vi "test_MSS simulated scope.vi"(8 "Error In":errorcluster) -> (0 "Error Out":errorcluster)   [LabVIEW 2023]
uses:
  Measure and Stimulus Subsystems/Measure and Stimulus Subsystems.lvclass
panel:
  out "Powersensor Chart":waveform(dbl)(graph)
  in  "Stop":bool
  out "Photosensor Chart":waveform(dbl)(graph)
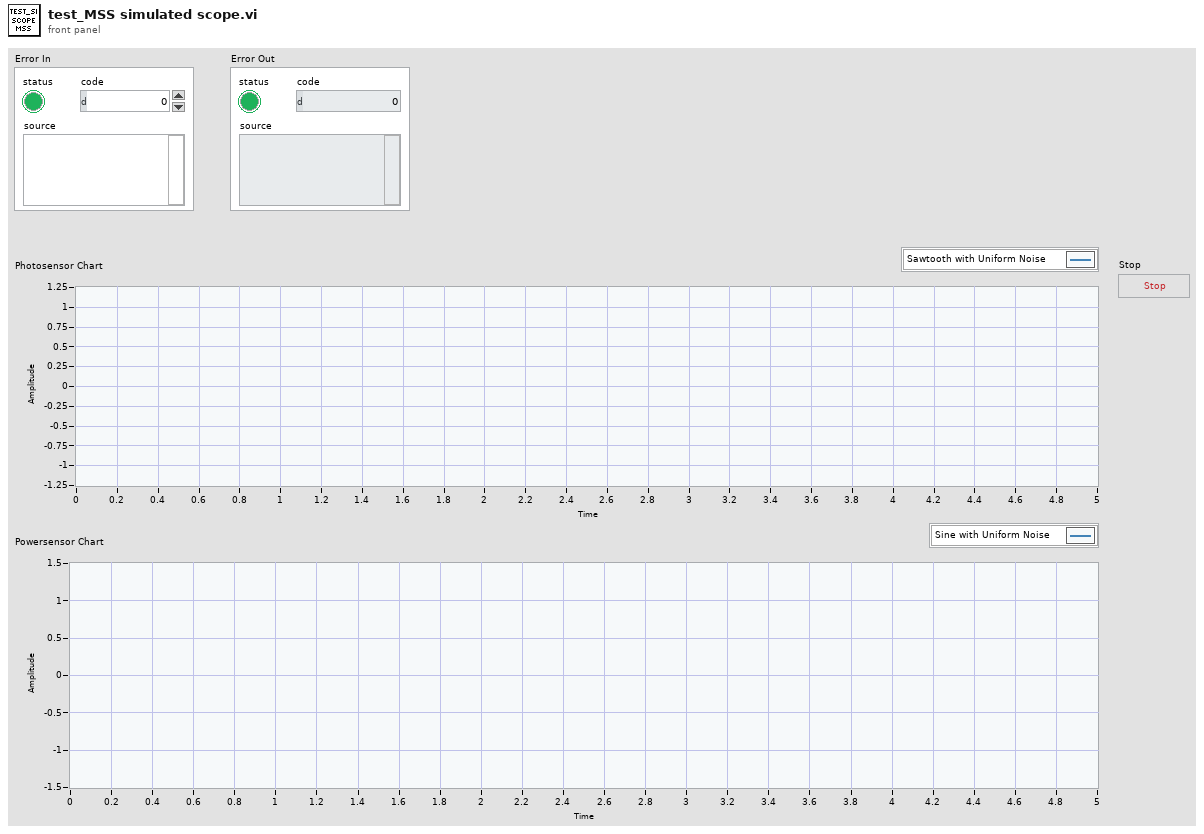
[diagram p1: front panel]
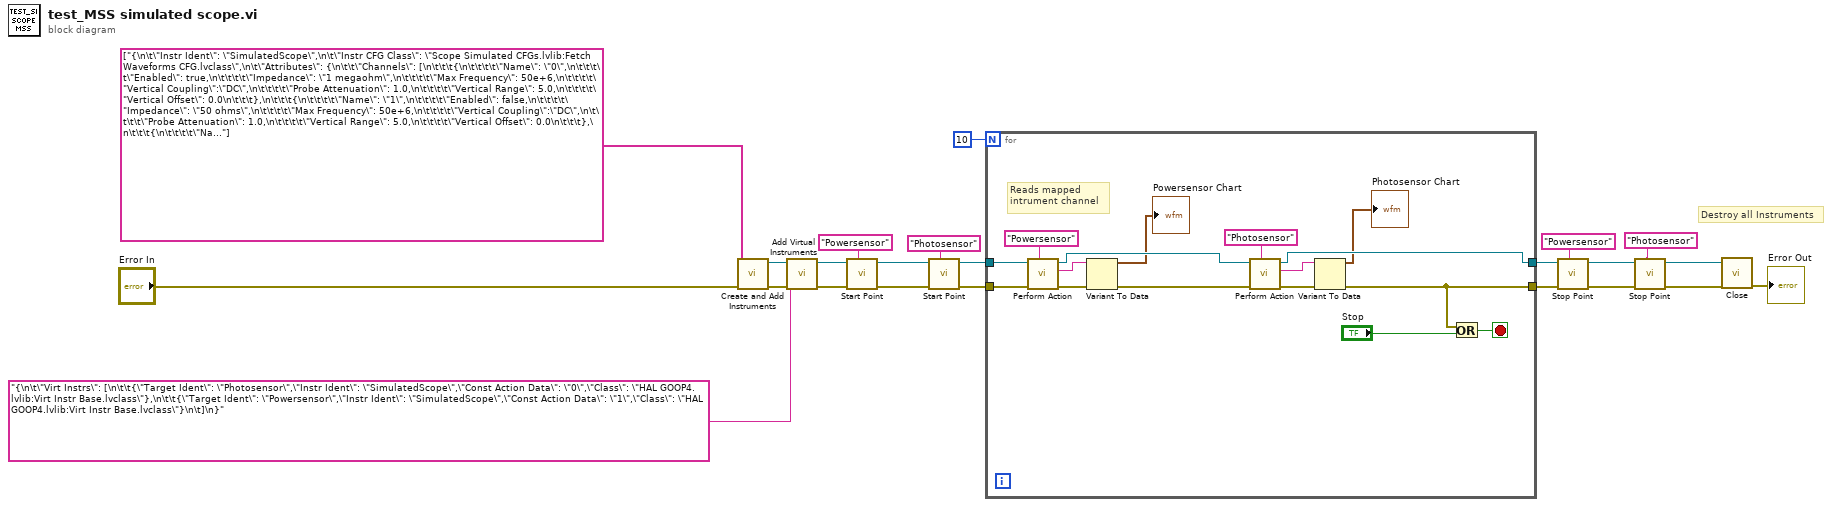
[diagram p0: block diagram]
diagram:
  # "Destroy all Instruments"
  n1 = call "Create and Add Instruments.vi"("Error In"="Error In", "Physical Intr CFGs"=string[] ["{\n\t\"Instr Ident\": \"SimulatedScope\",\n\t\"Instr CFG Class\": \"Scope Simulated CFGs.lvlib:Fetch Waveforms CFG.lvclass\",\n\t\"Attributes\": {\n\t\t\"Channels\": [\n\t\t\t{\n\t\t\t\t\"Name\": \"0\",\n\t\t\t\t\"Enabled\": true,\n\t\t\t\t\"Impedance\": \"1 megaohm\",\n\t\t\t\t\"Max Frequency\": 50e+6,\n\t\t\t\t\"Vertical Coupling\":\"DC\",\n\t\t\t\t\"Probe Attenuation\": 1.0,\n\t\t\t\t\"Vertical Range\": 5.0,\n\t\t\t\t\"Vertical Offset\": 0.0\n\t\t\t},\n\t\t\t{\n\t\t\t\t\"Name\": \"1\",\n\t\t\t\t\"Enabled\": false,\n\t\t\t\t\"Impedance\": \"50 ohms\",\n\t\t\t\t\"Max Frequency\": 50e+6,\n\t\t\t\t\"Vertical Coupling\":\"DC\",\n\t\t\t\t\"Probe Attenuation\": 1.0,\n\t\t\t\t\"Vertical Range\": 5.0,\n\t\t\t\t\"Vertical Offset\": 0.0\n\t\t\t},\n\t\t\t{\n\t\t\t\t\"Name\": \"2\",\n\t\t\t\t\"Enabled\": false,\n\t\t\t\t\"Impedance\": \"50 ohms\",\n\t\t\t\t\"Max Frequency\": 50e+6,\n\t\t\t\t\"Vertical Coupling\":\"DC\",\n\t\t\t\t\"Probe Attenuation\": 1.0,\n\t\t\t\t\"Vertical Range\": 5.0,\n\t\t\t\t\"Vertical Offset\": 0.0\n\t\t\t},\n\t\t\t{\n\t\t\t\t\"Name\": \"3\",\n\t\t\t\t\"Enabled\": true,\n\t\t\t\t\"Impedance\": \"50 ohms\",\n\t\t\t\t\"Max Frequency\": 50e+6,\n\t\t\t\t\"Vertical Coupling\":\"DC\",\n\t\t\t\t\"Probe Attenuation\": 1.0,\n\t\t\t\t\"Vertical Range\": 1.4,\n\t\t\t\t\"Vertical Offset\": 0.0\n\t\t\t},\n\t\t\t{\n\t\t\t\t\"Name\": \"4\",\n\t\t\t\t\"Enabled\": false,\n\t\t\t\t\"Impedance\": \"50 ohms\",\n\t\t\t\t\"Max Frequency\": 50e+6,\n\t\t\t\t\"Vertical Coupling\":\"DC\",\n\t\t\t\t\"Probe Attenuation\": 1.0,\n\t\t\t\t\"Vertical Range\": 5.0,\n\t\t\t\t\"Vertical Offset\": 0.0\n\t\t\t},\n\t\t\t{\n\t\t\t\t\"Name\": \"5\",\n\t\t\t\t\"Enabled\": false,\n\t\t\t\t\"Impedance\": \"50 ohms\",\n\t\t\t\t\"Max Frequency\": 50e+6,\n\t\t\t\t\"Vertical Coupling\":\"DC\",\n\t\t\t\t\"Probe Attenuation\": 1.0,\n\t\t\t\t\"Vertical Range\": 5.0,\n\t\t\t\t\"Vertical Offset\": 0.0\n\t\t\t},\n\t\t\t{\n\t\t\t\t\"Name\": \"6\",\n\t\t\t\t\"Enabled\": false,\n\t\t\t\t\"Impedance\": \"50 ohms\",\n\t\t\t\t\"Max Frequency\": 50e+6,\n\t\t\t\t\"Vertical Coupling\":\"DC\",\n\t\t\t\t\"Probe Attenuation\": 1.0,\n\t\t\t\t\"Vertical Range\": 5.0,\n\t\t\t\t\"Vertical Offset\": 0.0\n\t\t\t},\n\t\t\t{\n\t\t\t\t\"Name\": \"7\",\n\t\t\t\t\"Enabled\": false,\n\t\t\t\t\"Impedance\": \"50 ohms\",\n\t\t\t\t\"Max Frequency\": 50e+6,\n\t\t\t\t\"Vertical Coupling\":\"DC\",\n\t\t\t\t\"Probe Attenuation\": 1.0,\n\t\t\t\t\"Vertical Range\": 5.0,\n\t\t\t\t\"Vertical Offset\": 0.0\n\t\t\t}\n\t\t],\n\t\t\"Horizontal\": {\n\t\t\t\"Enforce Realtime\": true,\n\t\t\t\"Number of Records\": 1,\n\t\t\t\"Min Sample Rate\": 1e+5,\n\t\t\t\"Reference Position\":50, //percent\n\t\t\t\"Min Record Length\":1e+3\n\t\t},\n\t\t\"Acquire\": {\n\t\t\t\"Type\": \"Normal\",\n\t\t\t\"NumSamples\": 1e+3,\n\t\t\t\"Fetch Relative To\": \"Read Pointer\"\n\t\t},\n\t\t\"Export Signal\": {\n\t\t\t\"Signal Identifier\": \"None\",\n\t\t\t\"Signal\": \"None\",\n\t\t\t\"Output Terminal\": \"None\"\n\t\t},\n\t\t\"Trigger\": {\n\t\t\t\"Type\": \"Immediate\",\n\t\t\t\"Slope\": \"Positive\",\n\t\t\t\"Source\": \"RTSI 0\",\n\t\t\t\"Holdoff\": 0.0,\n\t\t\t\"Delay\": 0.0\n\t\t}\n\t}\n}"]) -> ("Error Out"=w20:errorcluster, "MSS out"=w5:refnum<class "Measure and Stimulus Subsystems.lvclass">)  [unwired: 7 in, 1 out]
  n2 = call "Add Virtual Instruments.vi"("error in"=w20, "<JSON CFG>"="{\n\t\"Virt Instrs\": [\n\t\t{\"Target Ident\": \"Photosensor\",\"Instr Ident\": \"SimulatedScope\",\"Const Action Data\": \"0\",\"Class\": \"HAL GOOP4.lvlib:Virt Instr Base.lvclass\"},\n\t\t{\"Target Ident\": \"Powersensor\",\"Instr Ident\": \"SimulatedScope\",\"Const Action Data\": \"1\",\"Class\": \"HAL GOOP4.lvlib:Virt Instr Base.lvclass\"}\n\t]\n}", "MSS in"=w5) -> ("error out"=w6:errorcluster, "MSS out"=w4:refnum<class "Measure and Stimulus Subsystems.lvclass">)  [unwired: 6 in, 1 out]
  n3 = call "Start Point.vi"("Point Ident"="Powersensor" ("Target Ident"), "error in"=w6, "MSS in"=w4) -> ("error out"=w18:errorcluster, "MSS out"=w16:refnum<class "Measure and Stimulus Subsystems.lvclass">)  [unwired: 7 in]
  n4 = call "Start Point.vi"("Point Ident"="Photosensor" ("Target Ident"), "error in"=w18, "MSS in"=w16) -> ("error out"=w17:errorcluster, "MSS out"=w15:refnum<class "Measure and Stimulus Subsystems.lvclass">)  [unwired: 7 in]
  n5 = for {
    N: 10 -> [_]
    tunnel: w17 -> [w32]
    tunnel: w15 -> [w31]
    tunnel: [w33] -> w11
    tunnel: [w35] -> w22
    stop <- w39 stop-if-true
    # "Reads mapped\nintrument channel"
    n6 = call "Perform Action.vi"("Task Ident"="Powersensor" ("Target Identifier"), "error in"=w32, "MSS in"=w31) -> ("error out"=w30:errorcluster, "Task-Point Ident"=w26:string, "MSS out"=w27:refnum<class "Measure and Stimulus Subsystems.lvclass">)  [unwired: 5 in, 1 out]
    n7 = Variant To Data(error in=w30, Variant=w26) -> (data=→"Powersensor Chart":waveform(dbl), error out=w28:errorcluster)  [unwired: 1 in]
    n8 = call "Perform Action.vi"("Task Ident"="Photosensor" ("Target Identifier"), "error in"=w28, "MSS in"=w27) -> ("error out"=w37:errorcluster, "Task-Point Ident"=w34:string, "MSS out"=w33:refnum<class "Measure and Stimulus Subsystems.lvclass">)  [unwired: 5 in, 1 out]
    n9 = Variant To Data(error in=w37, Variant=w34) -> (data=→"Photosensor Chart":waveform(dbl), error out=w35:errorcluster)  [unwired: 1 in]
    n10 = Or(x=w35, y="Stop") -> (x .or. y?=w39:bool)
  }
  n11 = call "Stop Point.vi"("Point Ident"="Powersensor" ("Target Ident"), "error in"=w22, "MSS in"=w11) -> ("error out"=w12:errorcluster, "MSS out"=w10:refnum<class "Measure and Stimulus Subsystems.lvclass">)  [unwired: 7 in]
  n12 = call "Stop Point.vi"("Point Ident"="Photosensor" ("Target Ident"), "error in"=w12, "MSS in"=w10) -> ("error out"=w1:errorcluster, "MSS out"=w2:refnum<class "Measure and Stimulus Subsystems.lvclass">)  [unwired: 7 in]
  n13 = call "Close.vi"("error in"=w1, "MSS in"=w2) -> ("error out"=→"Error Out":errorcluster)  [unwired: 8 in, 1 out]
